vi "systemConfigInitialisation.vi"(8 "configData":T3 {"allValues"."safetyLimits"."channelLimits"."channelID" items=["time", "gearbox", "compressor bearing", "shaft bearing", "oil outlet", "inlet 1", "inlet 2", "outlet 1", "outlet 2", "inlet pressure", "outlet pressure", "plenum pressure", "Motor speed", "new V-cone DP", "Motor power", "Accelerometer", "Hotwire 1", "oil pressure", "butterfly valve position", "ball valve position", "Legacy speed", "Torque speed", "pulsator encoder", "v-cone upstream 1", "v-cone upstream 2"]}) -> (0 "configData out":T3 {"allValues"."safetyLimits"."channelLimits"."channelID" items=["time", "gearbox", "compressor bearing", "shaft bearing", "oil outlet", "inlet 1", "inlet 2", "outlet 1", "outlet 2", "inlet pressure", "outlet pressure", "plenum pressure", "Motor speed", "new V-cone DP", "Motor power", "Accelerometer", "Hotwire 1", "oil pressure", "butterfly valve position", "ball valve position", "Legacy speed", "Torque speed", "pulsator encoder", "v-cone upstream 1", "v-cone upstream 2"]})   [LabVIEW 2018]
uses:
  systemConfigUIControls.ctl
  type defs/channelLimitControl.ctl
  type defs/limitActions.ctl
  ICL-LabVIEW_General/data channels/parent class/Data Channel.lvclass
  ICL-LabVIEW_General/data channels/parent class/channel type.ctl
  ICL-LabVIEW_General/data channels/parent class/Supporting functions/channel filter - type.vi
  ICL-LabVIEW_General/data channels/data channels.lvlib
panel:
  in  "channelLimit":T1
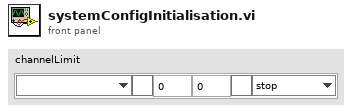
[diagram p1: front panel]
types:
  T1 = typedef "channelLimitControl.ctl" = cluster{"channelID":u16, "Enabled":bool, "warnValue":dbl, "limitValue":dbl, "Invert":bool, "limitAction":T2}
  T2 = typedef "limitActions.ctl" = enum16{"stop", "shutdown", "ignore"}
  T3 = typedef "systemConfigUIControls.ctl" = cluster{"allControls":cluster{"feedbackChannels":cluster{"butterfly":refnum<vi>, "ball":refnum<vi>, "massflow":refnum<vi>, "pressureRatio":refnum<vi>, "airP":refnum<vi>, "water":refnum<vi>, "oilP":refnum<vi>, "speed":refnum<vi>}, "controlChannels":cluster{"butterflyControl":refnum<vi>, "ballControl":refnum<vi>, "speedControl":refnum<vi>}, "channelLimits":refnum<vi>, "pulsatorIP":string}, "allValues":cluster{"feedback":cluster{"butterfly":u16, "ball":u16, "massflow":u16, "pressureRatio":u16, "airP":u16, "water":u16, "oilP":u16, "speed":u16}, "paths":cluster{"channelConfig":path, "systemConfig":path, "incidentLogfile":path, "startFolder":path, "customVI":path}, "RT":cluster{"RTIP":string, "errorReaderName":string, "errorWriterName":string, "errorBufferSize":u16, "commandWriterName":string, "commandReaderName":string, "commandBufferSize":u16, "dataBufferSize":u16, "dataReaderName":string, "dataWriterName":string, "dataBufferLength":u16, "scanivalveIP":string, "scanPeriod":u16}, "controls":cluster{"butterflyControl":u16, "ballControl":u16, "speedControl":u16}, "safetyLimits":cluster{"channelLimits":T1[], "maxSpeed":u32}, "Howden":cluster{"howdenAir":bool, "howden%":dbl}}, "variables":cluster{"feedbackChannelIDs":u16[], "controlChannelIDs":u16[], "channelsArray":refnum<class "Data Channel.lvclass">[]}}
  T4 = typedef "message handler data.ctl" = cluster{"params":cluster{"configFileID":u32, "configFilePath":path, "channelConfigFilePath":path, "incidentLogfile":path, "controlChannels":cluster{"ballControl":u16, "butterflyControl":u16, "speedControl":u16}, "pulsatorVIPath":path, "customVIPath":path, "HowdenAir":cluster{"vent Howden":bool, "Howden%":dbl}}, "vars":cluster{"commsStatus":bool[], "controlIndex":cluster{"ballControl":u16, "butterflyControl":u16, "speedControl":u16}, "customVIRef":refnum<vi>, "Interlocks":cluster{"gearboxOil":bool, "bearingOil":bool, "gearboxAir":bool}, "motorRunning":bool, "liveDataQ":refnum<queue>[]}}
  T5 = typedef "comms loop data.ctl" = cluster{"params":cluster{"commandStream":cluster{"reader name":string, "writer name":string, "stream buffer size":i32}, "errorStream":cluster{"reader name":string, "writer name":string, "stream buffer size":i32}, "RT IP address":string, "pulserControllerIP":string}, "vars":cluster{"commandStream":refnum<k21>, "Incident logger":refnum<class "Incident logger.lvclass">, "check error scheduled message":u32, "errorStream":refnum<k21>, "watchdogScheduleID":u32, "pulsator":cluster{"pulser connection":refnum<class "Modbus Master.lvclass">, "pulserConnected":bool, "pulsatorScheduleID":u32, "pulserRunning":bool}}}
  T6 = typedef "data stream data.ctl" = cluster{"params":cluster{"Stream":cluster{"reader name":string, "RT IP address":string, "writer name":string, "stream buffer size":i32}}, "vars":cluster{"data stream":refnum<k21>}}
  T7 = typedef "data processor data.ctl" = cluster{"params":cluster{"controlFeedback":cluster{"butterflyValue":u16, "ballValue":u16, "massflow":u16, "pressureRatio":u16, "compSpeed":u16}, "DAQrate":enum16{"50 kHz", "25 kHz", "16.6 kHz", "12.5 kHz", "10 kHz", "8.33 kHz", "7.14 kHz", "6.25 kHz", "5.55 kHz", "5 kHz"}, "safetyChannels":cluster{"oilP":u16, "airP":u16, "water":u16, "channelLimit":T1[]}, "channelConfigPath":path}, "vars":cluster{"controlFeedback":cluster{"butterflyValue":u16, "ballValue":u16, "massflow":u16, "pressureRatio":u16, "compSpeed":u16}, "activeChannelNames":string[], "activeChannelUnits":string[], "offset trigger":bool, "offsets":dbl[], "activeChannelLimitIndex":u16[], "liveData":bool}}
  T8 = typedef "file IO data.ctl" = cluster{"params":cluster{"startFolder":path, "channelConfigPath":path}, "vars":cluster{"channelConfig ":T9[], "writing":cluster{"streaming":bool, "fixedLength":bool, "pointCount":u32, "timeZero":dbl, "pointsWritten":u32, "dataRate":u16}, "channelCount":u16, "fileTarget":cluster{"Save folder":path, "Target filename":string, "file ref":refnum<file>, "pulsatorSpeed":string, "motorSpeed":string, "valvePosition":string, "torqueFilter":bool, "pulsatorRunning":bool, "motorRunning":bool}, "channels":refnum<class "Data Channel.lvclass">[]}}
  T9 = typedef "channelControl.ctl" = cluster{"index":u16, "active":bool, "channelType":T10, "module":u16, "terminal":u16, "channelName":string, "scalingMethod":T11, "scalingParameters":dbl[], "scaledUnits":string, "tempOffset":dbl}
  T10 = typedef "channelScalingTypes.ctl" = enum16{"calculation", "measurement", "scanivalve", "output", "digital"}
  T11 = typedef "scalingMethods.ctl" = enum16{"none", "linear", "thermocouple", "polynomial", "encoder", "RTD"}
  T12 = typedef "UI loop data.ctl" = cluster{"params":cluster{"channelConfigPath":path, "version":string}, "vars":cluster{"tempOffsets":dbl[], "encoderFallingEdge":bool, "controlRefs":cluster{"mainVI":refnum<vi>, "menu":refnum<k9>, "motorStart":refnum<vi>, "butterfly":refnum<vi>, "ball":refnum<vi>, "speed":refnum<vi>, "logLimit":refnum<vi>, "pointLimit":refnum<vi>, "logData":refnum<vi>}}}
  T13 = typedef "error messages data.ctl" = cluster{"params":cluster{"eg":bool}, "vars":cluster{"eg":bool}}
  T14 = cluster{"messageHandler":T4, "comms":T5, "dataStream":T6, "dataProcessor":T7, "fileIO":T8, "userInterface":T12, "errors":T13}
  T15 = typedef "data channels.lvlib/Data Channel.lvclass/channel type.ctl" = enum16{"acquisition", "output", "other"}
  T16 = typedef "Message loop data.ctl" = cluster{"Parameters":cluster{"FPGA Ref":T17, "configID":u32, "activeChannels":cluster{"index":u16, "name":string}[]}, "Variables":cluster{"RT Status":T18, "watchdog":timestamp, "limitsEnabled":bool, "Interlocks":cluster{"gearboxOil":bool, "bearingOil":bool, "gearboxAir":bool}}}
  T17 = typedef "FPGA reference.ctl" = refnum<k20>
  T18 = typedef "RT Status.ctl" = cluster{"Comms loop":bool, "scheduler loop":bool, "data process loop":bool, "FIFO loop":bool, "Command Stream":bool, "Error Stream":bool, "FPGA FIFO":bool, "Data Stream":bool}
  T19 = typedef "Analogue loop data.ctl" = cluster{"Params":cluster{"FPGA ref":T17, "Total Channels":u32}, "Variables":cluster{"FIFO wait counter":u16, "FIFO read trigger":u32}}
  T20 = typedef "comms data.ctl" = cluster{"Parameters":cluster{"error writer name":string, "command reader name":string, "error buffer size":i32, "command buffer size":i32, "scanivalveIP":string, "scanivalvePeriod":u16}, "Variables":cluster{"listen schedule":u32, "incident buffer":T21[], "command stream":refnum<k21>, "error stream":refnum<k21>, "waiting for command stream connect":bool, "waiting for error stream connect":bool, "scanivalve connection":refnum<k5>, "scanivalveScheduleID":u32, "activeScanivalvePorts":i32[], "channelCount":i16}, "scanivalveConfig":T22}
  T21 = typedef "generic incident.ctl" = cluster{"timestamp":timestamp, "type":string, "Variant":variant}
  T22 = typedef "Scanivalve API.lvlib/scanivalveConfig.ctl" = cluster{"listS":T23, "listC":T24, "listSG":T25, "activeChannels":T26}
  T23 = typedef "Scanivalve API.lvlib/listS.ctl" = cluster{"period":u16, "ADtrig":bool, "ScanTrig":bool, "page":u16, "qpkts":u16}
  T24 = typedef "Scanivalve API.lvlib/listC.ctl" = cluster{"ZC":bool, "unitScan":string, "CvtUnit":dbl, "bin":bool, "EU":bool}
  T25 = typedef "Scanivalve API.lvlib/listSG.ctl" = cluster{"Avg1":u16, "FPS1":u16, "SGEnable1":bool}
  T26 = typedef "Scanivalve API.lvlib/chan1.ctl" = cluster{"Chan1":cluster{"101":bool, "102":bool, "103":bool, "104":bool, "109":bool, "110":bool, "111":bool, "112":bool, "201":bool, "202":bool, "203":bool, "204":bool, "209":bool, "210":bool, "211":bool, "212":bool, "301":bool, "302":bool, "303":bool, "304":bool, "309":bool, "310":bool, "311":bool, "312":bool, "401":bool, "402":bool, "403":bool, "404":bool, "409":bool, "410":bool, "411":bool, "412":bool}}
  T27 = typedef "Data processing loop data.ctl" = cluster{"Parameters":cluster{"FPGA Ref":T17, "data stream":cluster{"data writer name":string, "NS write buffer size":i32, "NS Buffer length":u32}, "FIFO Depth":u32, "Channel controls":cluster{"FIFO channel count":i32, "active indices":i16[], "active channels":i32, "channelScaling":T9[], "scanivalveCount":i32, "channels":refnum<class "Data Channel.lvclass">[]}, "safetyChannels":cluster{"oilP":u16, "airP":u16, "water":u16, "channelLimits":T1[]}, "speedChannel":i32, "maxSpeedLimit":dbl, "Torque":cluster{"fixedOffset":dbl, "filter":bool, "fallingEdge":bool, "swapEncoders":bool}}, "Variables":cluster{"Intermediary buffer":dbl[][], "buffer position":u32, "write loop counter":u16, "NS write trigger":u32, "NS Connection status":bool, "waiting for NS":bool, "labAmbient":cluster{"pressure":dbl, "temperature":dbl}, "scanivalvePorts":u16[], "scanivalvePressures":dbl[], "data stream":refnum<k21>, "activeChannelLimitIndex":u16[], "runningSpeedLimit":dbl, "speedChannelIndex":i32, "Interlocks":cluster{"gearboxOil":bool, "bearingOil":bool, "gearboxAir":bool}, "interlockChannels":cluster{"gearboxOil":i32, "bearingOil":i32, "air":i32}, "limitStates":cluster{"warn":bool, "alarm":bool}[]}}
  T28 = cluster{"Message":T16, "FIFO":T19, "Comms data":T20, "Data processor":T27}
  T29 = cluster{"butterfly":refnum<vi>, "ball":refnum<vi>, "massflow":refnum<vi>, "pressureRatio":refnum<vi>, "airP":refnum<vi>, "water":refnum<vi>, "oilP":refnum<vi>, "speed":refnum<vi>}
  T30 = cluster{"butterflyControl":refnum<vi>, "ballControl":refnum<vi>, "speedControl":refnum<vi>}
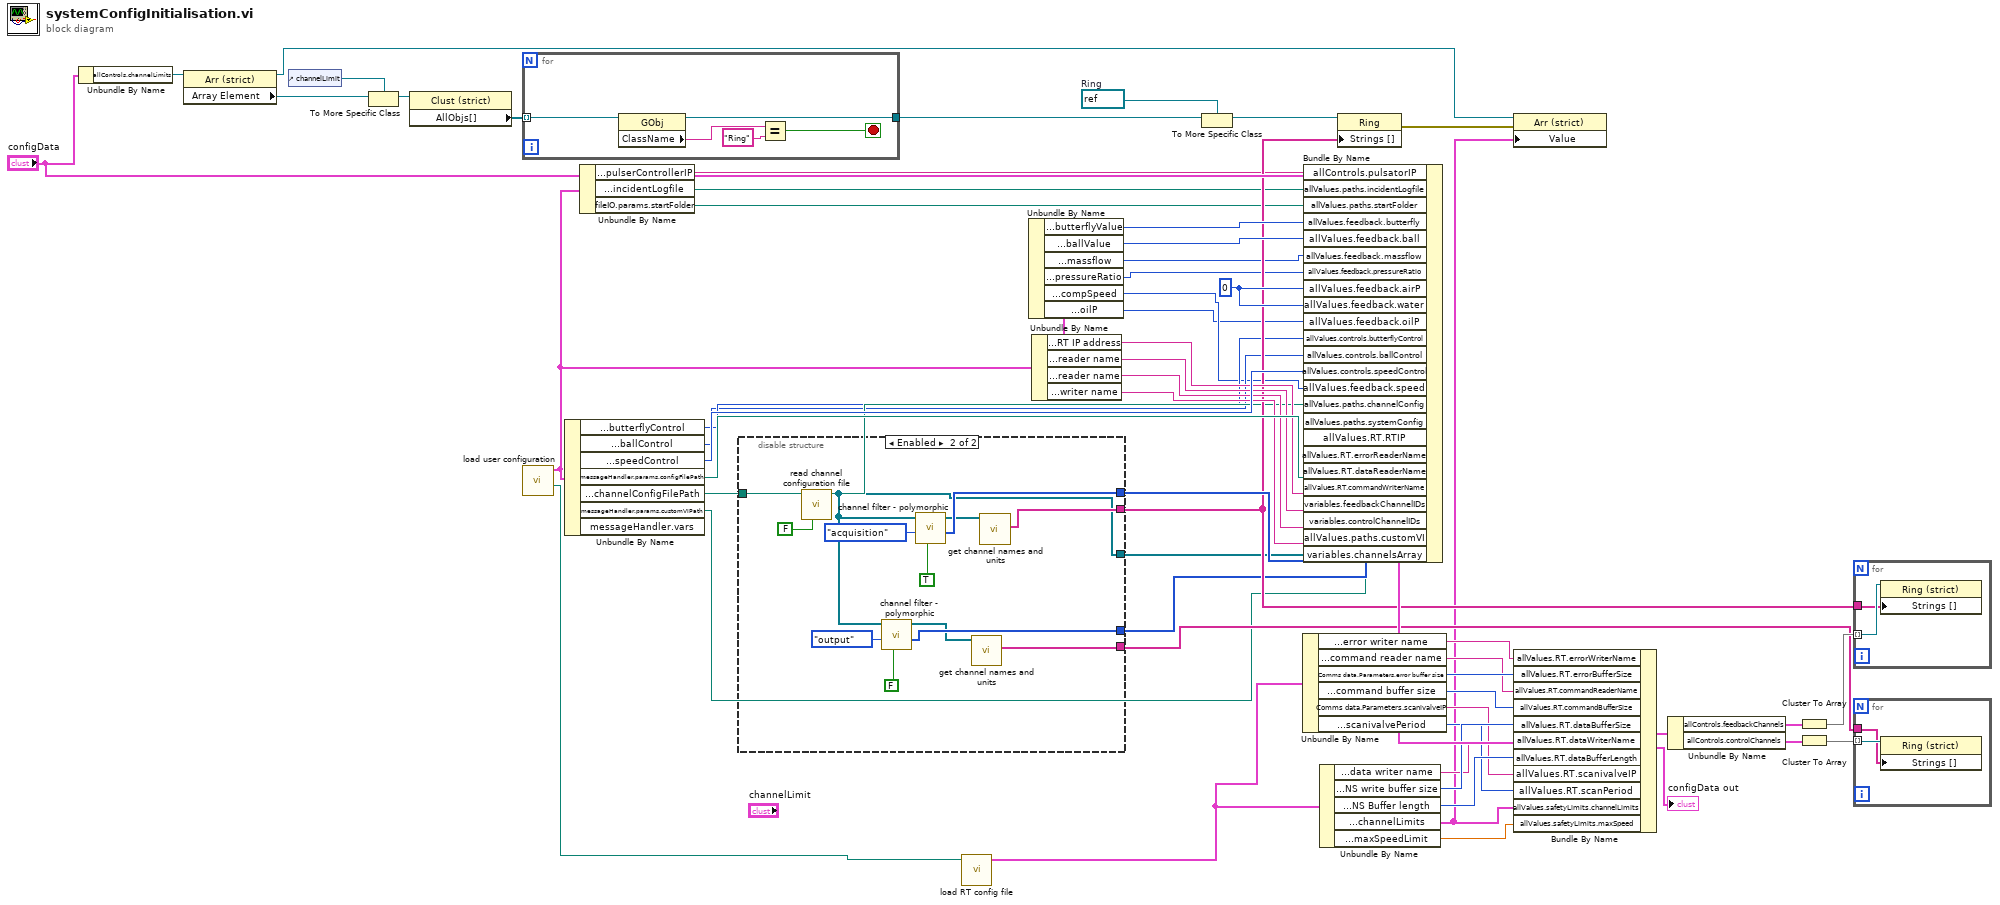
[diagram p0: block diagram]
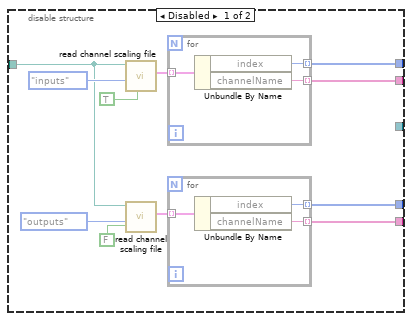
[diagram p2: hidden frame]
diagram:
  w38 = u16 0 ("allValues.channelValues.airP")
  w56 = refnum<vi> refnum  # Ring
  n1 = Unbundle By Name("configData") -> ("allControls.channelLimits"=w40:refnum<vi>)
  n2 = property class="Arr (strict)"(reference=w40) -> (reference out=w12:refnum<vi>, "Array Element"=w54:refnum<vi>)  [unwired: 1 in, 1 out]
  n3 = control-ref of="channelLimit"() -> (w42:refnum<vi>)
  n4 = To More Specific Class(target class=w42, reference=w54) -> (specific class reference=w55:refnum<vi>)  [unwired: 1 in, 1 out]
  n5 = property class="Clust (strict)"(reference=w55) -> ("AllObjs[]"=w37:refnum<vi>[])  [unwired: 1 in, 2 out]
  n6 = for {
    tunnel: w37 -> [w61] mode=indexing
    tunnel: [w57] -> w36
    stop <- w58 stop-if-true
    n7 = property class="GObj"(reference=w61) -> (reference out=w57:refnum<vi>, "ClassName"=w60:string)  [unwired: 1 in, 1 out]
    n8 = Equal?(x=w60, y="Ring") -> (x = y?=w58:bool)
  }
  n9 = call "load user configuration.vi"() -> ("RT config file path"=w8:path, "config parameters"=w26:T14)  [unwired: 10 in]
  n10 = Unbundle By Name(w26) -> ("messageHandler.params.controlChannels.butterflyControl"=w28:u16, "messageHandler.params.controlChannels.ballControl"=w27:u16, "messageHandler.params.controlChannels.speedControl"=w53:u16, "messageHandler.params.configFilePath"=w50:path, "messageHandler.params.channelConfigFilePath"=w33:path, "messageHandler.params.customVIPath"=w10:path)  [unwired: 1 out]
  n11 = Unbundle By Name(w26) -> ("comms.params.pulserControllerIP"=w2:string, "messageHandler.params.incidentLogfile"=w25:path, "fileIO.params.startFolder"=w24:path)
  n12 = disable-structure shown="Enabled" {
    disable-tunnel: [w69 w85] -> w35
    disable-tunnel: [w68 w83] -> w34
    disable-tunnel: w33 -> [w64 w91]
    disable-tunnel: [w63 w82] -> w30
    disable-tunnel: [w62 w88] -> w29
    disable-tunnel: [_ w80] -> w4
    frame Disabled {
      n13 = call "read channel scaling file.vi"("suppress inactive? (F)"=TRUE, "mode (all)"=enum16{"all", "inputs", "outputs", "digital"}."inputs", "file path"=w64) -> ("channelConfig"=w70:T9[])  [unwired: 4 in, 4 out]
      n14 = call "read channel scaling file.vi"("suppress inactive? (F)"=FALSE, "mode (all)"=enum16{"all", "inputs", "outputs", "digital"}."outputs", "file path"=w64) -> ("channelConfig"=w67:T9[])  [unwired: 4 in, 4 out]
      n15 = for {
        tunnel: w70 -> [w78] mode=indexing
        tunnel: [w77] -> w68 mode=indexing
        tunnel: [w76] -> w69 mode=indexing
        n16 = Unbundle By Name(w78) -> ("index"=w76:u16, "channelName"=w77:string)
      }
      n17 = for {
        tunnel: w67 -> [w75] mode=indexing
        tunnel: [w74] -> w63 mode=indexing
        tunnel: [w73] -> w62 mode=indexing
        n18 = Unbundle By Name(w75) -> ("index"=w73:u16, "channelName"=w74:string)
      }
    }
    frame Enabled {
      n19 = call "read channel configuration file.vi"("Hide inactive (F)"=FALSE, "config file"=w91) -> ("channelsArray"=w80:refnum<class "Data Channel.lvclass">[])  [unwired: 7 in, 2 out]
      n20 = call-poly "channel filter - polymorphic.vi"("activeOnly (F)"=FALSE, "channelType"=channel_type."output", "channels"=w80) -> ("filteredIndex"=w88:u16[], "filteredChannels"=w81:refnum<class "Data Channel.lvclass">[])  [unwired: 6 in, 1 out]
      n21 = call-poly "channel filter - polymorphic.vi"("activeOnly (F)"=TRUE, "channelType"=channel_type."acquisition", "channels"=w80) -> ("filteredIndex"=w85:u16[], "filteredChannels"=w84:refnum<class "Data Channel.lvclass">[])  [unwired: 6 in, 1 out]
      n22 = call "get channel names and units.vi"("channels"=w81) -> ("channelName"=w82:string[])  [unwired: 7 in, 3 out]
      n23 = call "get channel names and units.vi"("channels"=w84) -> ("channelName"=w83:string[])  [unwired: 7 in, 3 out]
    }
  }
  n24 = call "load RT config file.vi"("configuration file path (RT local)"=w8) -> ("config data out"=w9:T28)  [unwired: 7 in, 3 out]
  n25 = Unbundle By Name(w26) -> ("dataProcessor.params.controlFeedback.butterflyValue"=w52:u16, "dataProcessor.params.controlFeedback.ballValue"=w51:u16, "dataProcessor.params.controlFeedback.massflow"=w7:u16, "dataProcessor.params.controlFeedback.pressureRatio"=w6:u16, "dataProcessor.params.controlFeedback.compSpeed"=w5:u16, "dataProcessor.params.safetyChannels.oilP"=w3:u16)
  n26 = Unbundle By Name(w26) -> ("comms.params.RT IP address"=w49:string, "comms.params.errorStream.reader name"=w48:string, "dataStream.params.Stream.reader name"=w47:string, "comms.params.commandStream.writer name"=w46:string)
  n27 = To More Specific Class(target class=w56, reference=w36) -> (specific class reference=w39:refnum<vi>)  [unwired: 1 in, 1 out]
  n28 = Unbundle By Name(w9) -> ("Comms data.Parameters.error writer name"=w22:string, "Comms data.Parameters.command reader name"=w20:string, "Comms data.Parameters.error buffer size"=w21:i32, "Comms data.Parameters.command buffer size"=w19:i32, "Comms data.Parameters.scanivalveIP"=w15:string, "Comms data.Parameters.scanivalvePeriod"=w16:u16)
  n29 = Bundle By Name(cluster="configData", "allControls.pulsatorIP"=w2, "allValues.paths.incidentLogfile"=w25, "allValues.paths.startFolder"=w24, "allValues.feedback.butterfly"=w52, "allValues.feedback.ball"=w51, "allValues.feedback.massflow"=w7, "allValues.feedback.pressureRatio"=w6, "allValues.feedback.airP"=w38, "allValues.feedback.water"=w38, "allValues.feedback.oilP"=w3, "allValues.controls.butterflyControl"=w28, "allValues.controls.ballControl"=w27, "allValues.controls.speedControl"=w53, "allValues.feedback.speed"=w5, "allValues.paths.channelConfig"=w33, "allValues.paths.systemConfig"=w50, "allValues.RT.RTIP"=w49, "allValues.RT.errorReaderName"=w48, "allValues.RT.dataReaderName"=w47, "allValues.RT.commandWriterName"=w46, "variables.feedbackChannelIDs"=w35, "variables.controlChannelIDs"=w29, "allValues.paths.customVI"=w10, "variables.channelsArray"=w4) -> (w45:T3)
  n30 = Unbundle By Name(w9) -> ("Data processor.Parameters.data stream.data writer name"=w14:string, "Data processor.Parameters.data stream.NS write buffer size"=w18:i32, "Data processor.Parameters.data stream.NS Buffer length"=w17:u32, "Data processor.Parameters.safetyChannels.channelLimits"=w11:T1[], "Data processor.Parameters.maxSpeedLimit"=w1:dbl)
  n31 = property class="Ring"(reference=w39, "Strings []"=w34) -> (error out=w13:errorcluster)  [unwired: 1 in, 1 out]
  n32 = property class="Arr (strict)"(reference=w12, error in=w13, "Value"=w11) -> ()  [unwired: 2 out]
  n33 = Bundle By Name(cluster=w45, "allValues.RT.errorWriterName"=w22, "allValues.RT.errorBufferSize"=w21, "allValues.RT.commandReaderName"=w20, "allValues.RT.commandBufferSize"=w19, "allValues.RT.dataBufferSize"=w18, "allValues.RT.dataWriterName"=w14, "allValues.RT.dataBufferLength"=w17, "allValues.RT.scanivalveIP"=w15, "allValues.RT.scanPeriod"=w16, "allValues.safetyLimits.channelLimits"=w11, "allValues.safetyLimits.maxSpeed"=w1) -> (w23:T3)
  "configData out" <- w23
  n34 = Unbundle By Name(w23) -> ("allControls.feedbackChannels"=w44:T29, "allControls.controlChannels"=w32:T30)
  n35 = Cluster To Array(cluster=w44) -> (array=w43:refnum<vi>[])
  n36 = Cluster To Array(cluster=w32) -> (array=w31:refnum<vi>[])
  n37 = for {
    tunnel: w43 -> [w93] mode=indexing
    tunnel: w34 -> [w92]
    n38 = property class="Ring (strict)"(reference=w93, "Strings []"=w92) -> ()  [unwired: 1 in, 2 out]
  }
  n39 = for {
    tunnel: w31 -> [w95] mode=indexing
    tunnel: w30 -> [w94]
    n40 = property class="Ring (strict)"(reference=w95, "Strings []"=w94) -> ()  [unwired: 1 in, 2 out]
  }
